vi "Set Retardance (No Objects).vi"(8 "errorIN":errorcluster caption="Error", 9 "milliseconds to wait (0)":u32, 10 "Retardance":dbl[unit], 11 "Cluster In":T1) -> (0 "errorOUT":errorcluster caption="Error out", 2 "Retardance out":dbl[unit], 3 "Cluster Out":T1)   [LabVIEW 2017]
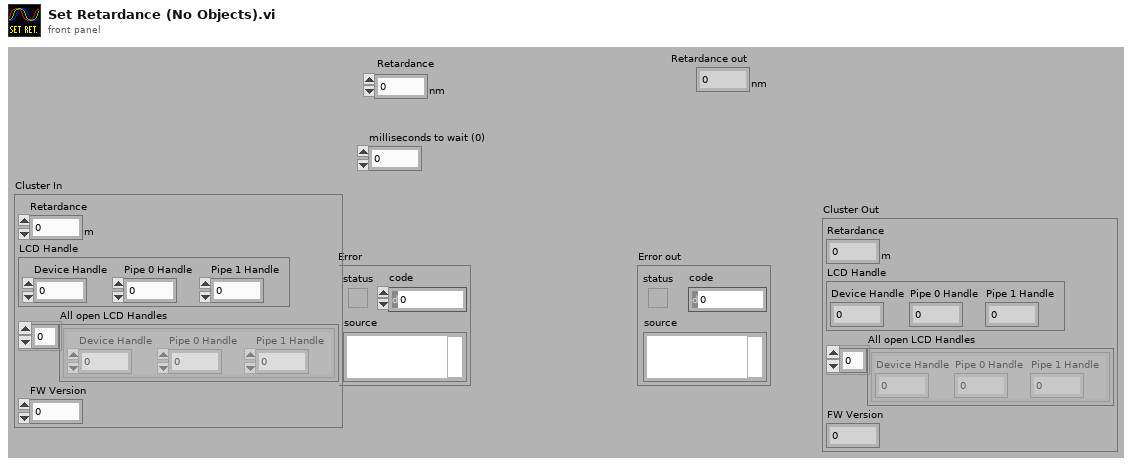
[diagram p1: front panel]
types:
  T1 = cluster{"Retardance":dbl[unit], "LCD Handle":cluster{"Device Handle":u32, "Pipe 0 Handle":u32, "Pipe 1 Handle":u32}, "All open LCD Handles":cluster{"Device Handle":u32, "Pipe 0 Handle":u32, "Pipe 1 Handle":u32}[], "FW Version":dbl}
  T2 = cluster{"Device Handle":u32, "Pipe 0 Handle":u32, "Pipe 1 Handle":u32}
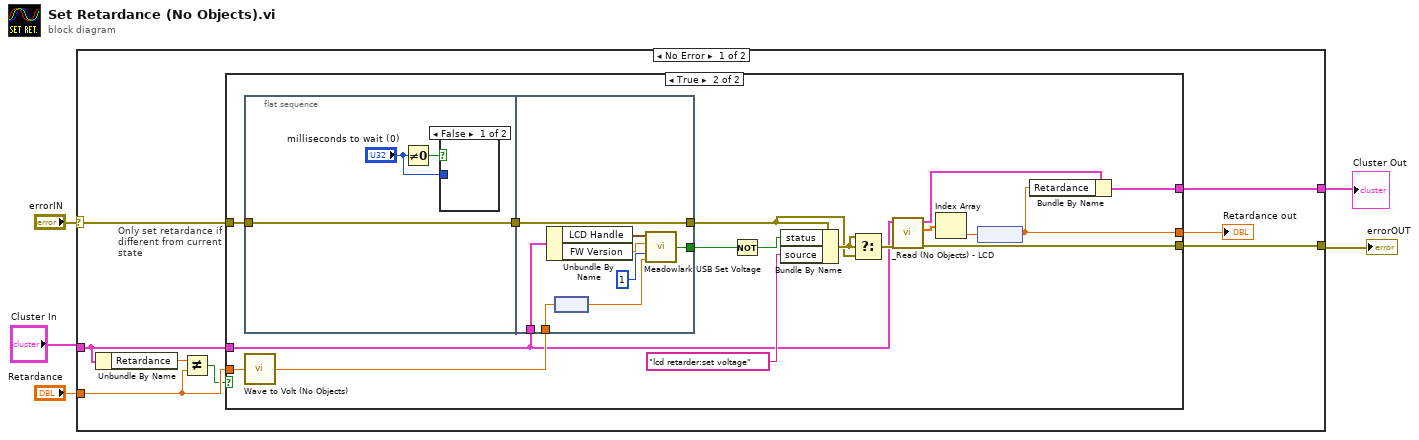
[diagram p0: block diagram]
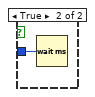
[diagram p3: hidden frame]
diagram:
  n1 = case shown="No Error" "errorIN" {
    selector: "errorIN" -> [w12 w46]
    tunnel: "Retardance" -> [w9 _]
    tunnel: "Cluster In" -> [w10 w47]
    tunnel: [w11 w47] -> w1
    tunnel: [w13 w46] -> w3
    frame No Error {
      n2 = Unbundle By Name(w10) -> ("Retardance"=w8:dbl[unit])
      n3 = Not Equal?(x=w8, y=w9) -> (x != y?=w7:bool)
      n4 = case "Only set retardance if different from current state" shown="True" w7 {
        tunnel: [w15 w31] -> w13
        tunnel: w12 -> [w15 w25]
        tunnel: [w16 w23] -> w11
        tunnel: w9 -> [w14 w21]
        tunnel: w10 -> [w16 w17]
        tunnel: [w14 w18] -> w6
        frame False {
          # "Only set retardance if different from current state"
        }
        frame True {
          n5 = flat-sequence {
            tunnel: w25 -> [w36]
            tunnel: [w36] -> w33
            tunnel: [w45] -> w26
            tunnel: w33 -> [w45]
            tunnel: w17 -> [w40]
            tunnel: w20 -> [w39]
            tunnel: [w38] -> w24
            frame #0 {
              n6 = Not Equal To 0?(x="milliseconds to wait (0)") -> (x != 0?=w34:bool)
              n7 = case shown="False" w34 {
                tunnel: "milliseconds to wait (0)" -> [_ w37]
                frame False {
                }
                frame True {
                  n8 = Wait (ms)(milliseconds to wait=w37) -> ()  [unwired: 1 out]
                }
              }
            }
            frame #1 {
              n9 = Unbundle By Name(w40) -> ("LCD Handle"=w43:T2, "FW Version"=w42:dbl)
              n10 = node(w39) -> (w44:dbl)
              n11 = call "Meadowlark USB Set Voltage.VI"("LC Voltage"=w44, "LC Channel"=1, "FW Version"=w42, "USB Open Device Cluster"=w43) -> ("Successful?"=w38:bool)
            }
          }
          n12 = call "Wave to Volt (No Objects).vi"("Retardance"=w21) -> ("Voltage"=w20:dbl[unit])
          n13 = Not(x=w24) -> (.not. x?=w30:bool)
          n14 = Bundle By Name(cluster=w26, "status"=w30, "source"="lcd retarder:set voltage") -> (w29:errorcluster)
          n15 = Select(t=w29, s=w29, f=w26) -> (s? t:f=w28:errorcluster)
          n16 = call "_Read (No Objects) - LCD.vi"("errorIN"=w28, "Cluster In"=w17) -> ("errorOUT"=w31:errorcluster, "X array"=w22:dbl[], "Cluster Out"=w32:T1)  [unwired: 7 in]
          n17 = Index Array(array=w22) -> (element=w19:dbl)  [unwired: 1 in]
          n18 = node(w19) -> (w18:dbl[unit])
          n19 = Bundle By Name(cluster=w32, "Retardance"=w18) -> (w23:T1)
        }
      }
      "Retardance out" <- w6
    }
    frame Error {
    }
  }
  "errorOUT" <- w3
  "Cluster Out" <- w1
